vi "Get Json Wfm Config.vi"(8 "error in":errorcluster, 11 "Json String":string) -> (0 "error out":errorcluster, 1 "Arbitrary Wfm Config":T1={"File Path"="", "Sample Rate (Hz)"=0.0, "Read From"=0, "Pre Delay (s)"=0.0, "Post Delay (s)"=0.0, "Scale"=1.0} {"Scale" min=0.0 format="%#_6p"}, 2 "Std Wfm Config":T2, 3 "Type":string(combo))   [LabVIEW 2025, in "TDMS Waveform Creator.lvclass"]
uses:
  <vilib>/Utility/error.llb/Error Cluster From Error Code.vi
  <vilib>/ErrorRing/Error Ring.xnode
  TDMS Waveform Creator.lvclass
  TDMS Waveform Creator.lvclass/TDMS Waveform Creator.ctl
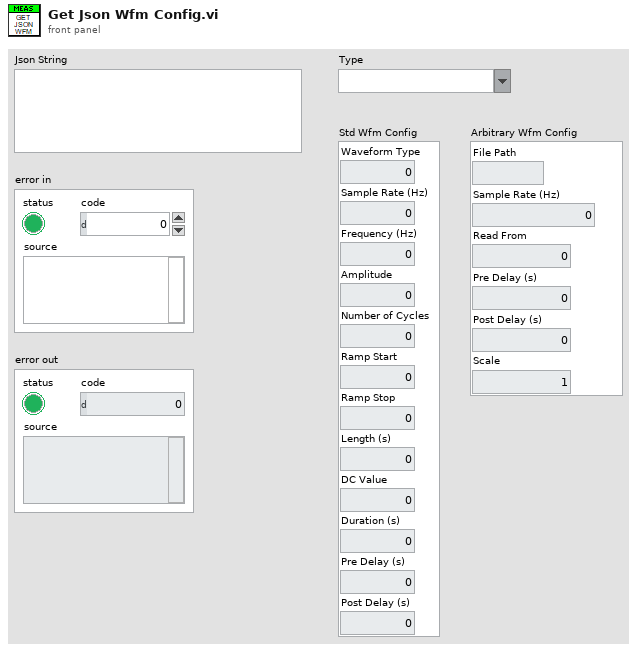
[diagram p1: front panel]
types:
  T1 = cluster{"File Path":string, "Sample Rate (Hz)":dbl, "Read From":i32, "Pre Delay (s)":dbl, "Post Delay (s)":dbl, "Scale":dbl}
  T2 = cluster{"Waveform Type":i32, "Sample Rate (Hz)":dbl, "Frequency (Hz)":dbl, "Amplitude":dbl, "Number of Cycles":u32, "Ramp Start":dbl, "Ramp Stop":dbl, "Length (s)":dbl, "DC Value":dbl, "Duration (s)":dbl, "Pre Delay (s)":dbl, "Post Delay (s)":dbl}
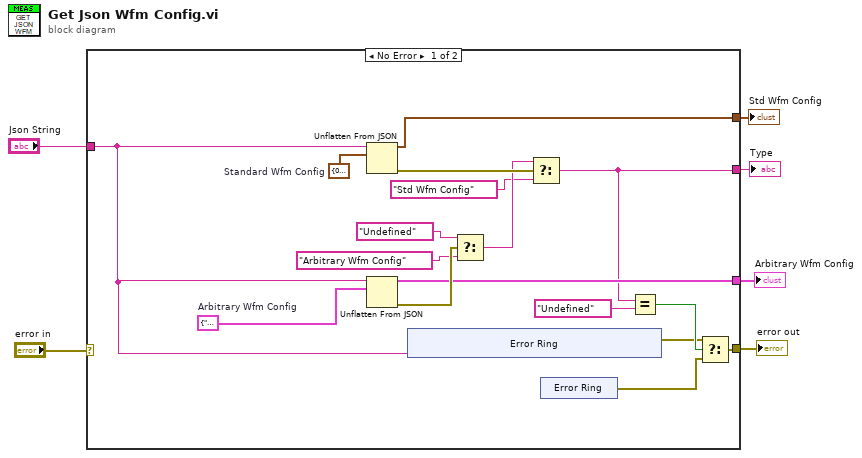
[diagram p0: block diagram]
diagram:
  n1 = case shown="No Error" "error in" {
    selector: "error in" -> [_ w32]
    tunnel: [w17 _] -> w6
    tunnel: [w16 _] -> w5
    tunnel: [w15 _] -> w4
    tunnel: "Json String" -> [w14 _]
    tunnel: [w10 w32] -> w2
    frame No Error {
      w22 = T2 {"Waveform Type"=0, "Sample Rate (Hz)"=10000000.0, "Frequency (Hz)"=0.0, "Amplitude"=0.0, "Number of Cycles"=0, "Ramp Start"=0.0, "Ramp Stop"=1.0, "Length (s)"=0.001, "DC Value"=0.0, "Duration (s)"=0.001, "Pre Delay (s)"=0.0, "Post Delay (s)"=0.0}  # Standard Wfm Config
      w23 = T1 {"File Path"="", "Sample Rate (Hz)"=10000000.0, "Read From"=10000, "Pre Delay (s)"=1.0, "Post Delay (s)"=1.0, "Scale"=1.0}  # Arbitrary Wfm Config
      n2 = Unflatten From JSON(JSON string=w14, type and defaults=w22) -> (value=w17:T2, error out=w20:errorcluster)  [unwired: 5 in]
      n3 = Unflatten From JSON(JSON string=w14, type and defaults=w23) -> (value=w16:T1, error out=w21:errorcluster)  [unwired: 5 in]
      n4 = xnode "Error Ring"("parameter 0"=w14) -> ("error out"=w12:errorcluster)
      n5 = Select(t="Undefined" ("Type"), s=w21, f="Arbitrary Wfm Config" ("Type")) -> (s? t:f=w19:string)
      n6 = Select(t=w19, s=w20, f="Std Wfm Config" ("Type")) -> (s? t:f=w15:string)
      n7 = xnode "Error Ring"() -> ("error out"=w11:errorcluster)
      n8 = Equal?(x=w15, y="Undefined" ("Type")) -> (x = y?=w13:bool)
      n9 = Select(t=w12, s=w13, f=w11) -> (s? t:f=w10:errorcluster)
    }
    frame Error {
    }
  }
  "Std Wfm Config" <- w6
  "Arbitrary Wfm Config" <- w5
  "Type" <- w4
  "error out" <- w2
